vi "_Main.vi"   [LabVIEW 2017, in "Joystick.lvlib"]
uses:
  Joystick.lvlib
  TypeDef Share All/ENUM_Joystick_Buttons.ctl
  TypeDef Share All/ENUM_Joystick_Axes.ctl
types:
  T1 = typedef "ENUM_Joystick_Axes.ctl" = enum16{"Left X", "Left Y", "Left Trigger", "Right Trigger", "Right X", "Right Y"}
  T2 = typedef "ENUM_Joystick_Buttons.ctl" = enum16{"Green A", "Red B", "Blue X", "Yellow Y", "Left Bumper", "Right Bumper", "Back", "Start", "Left Joystick", "Right Joystick"}
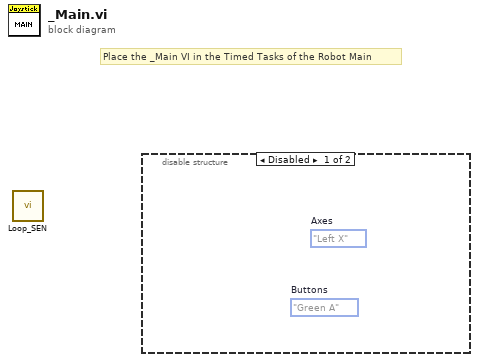
[diagram p0: block diagram]
diagram:
  # "Place the _Main VI in the Timed Tasks of the Robot Main"
  n1 = call "Loop_SEN.vi"() -> ()  [unwired: 12 in]
  n2 = disable-structure shown="Disabled" {
    frame Disabled {
      (unwired) ENUM_Joystick_Axes."Left X"  # Axes
      (unwired) ENUM_Joystick_Buttons."Green A"  # Buttons
    }
    frame Enabled {
    }
  }
